vi "Init Drone.vi"() -> (1 "Video Interface":refnum<k16>, 2 "NavData Port":refnum<k16>, 3 "AT Command Port":refnum<k16>)   [LabVIEW 2011]
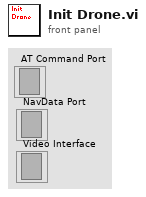
[diagram p1: front panel]
types:
  T1 = cluster{"Drone Status Bits":cluster{"Flying?":bool, "Video Enabled?":bool, "Vision Enabled?":bool, "Angular Speed Control?":bool, "Altitude Control?":bool, "Start button?":bool, "Control Command Recieved?":bool, "Trim Command Recieved?":bool, "Trim Running?":bool, "Trim Succeeded?":bool, "Navdata Demo Mode?":bool, "Navdata Bootstrap Mode?":bool, "Motors Com Down?":bool, "Unknown":bool, "Gyrometer Problem?":bool, "Battery Voltage Too Low?":bool, "Battery Voltage Too High?":bool, "Timer Elapsed?":bool, "Power Too Low?":bool, "Angles Out Of Range?":bool, "Too Much Wind?":bool, "Ultrasound Deaf?":bool, "Cutout Detected?":bool, "PIC Version Number OK?":bool, "ATCodec Thread On?":bool, "Navdata Thread On?":bool, "Video Thread On?":bool, "Acquisition Thread On?":bool, "Control Watchdog Delay?":bool, "ADC Watchdog Delay?":bool, "Communications Problem?":bool, "Emergency?":bool}, "Header":u32, "Sequence Number":u32, "Vision Defined?":bool, "Blocks":cluster{"Size":u16, "Data":u8[], "ID":enum16{"NAVDATA_DEMO", "NAVDATA_TIME", "NAVDATA_RAW_MEASURES", "NAVDATA_PHYS_MEASURES", "NAVDATA_GYROS_OFFSETS", "NAVDATA_EULER_ANGLES", "NAVDATA_REFERENCES", "NAVDATA_TRIMS", "NAVDATA_RC_REFERENCES", "NAVDATA_PWM", "NAVDATA_ALTITUDE", "NAVDATA_VISION_RAW", "NAVDATA_VISION_OF", "NAVDATA_VISION", "NAVDATA_VISION_PERF", "NAVDATA_TRACKERS_SEND", "NAVDATA_VISION_DETECT", "NAVDATA_WATCHDOG", "NAVDATA_ADC_DATA_FRAME", "NAVDATA_VIDEO_STREAM", "NAVDATA_GAMES"}}[]}
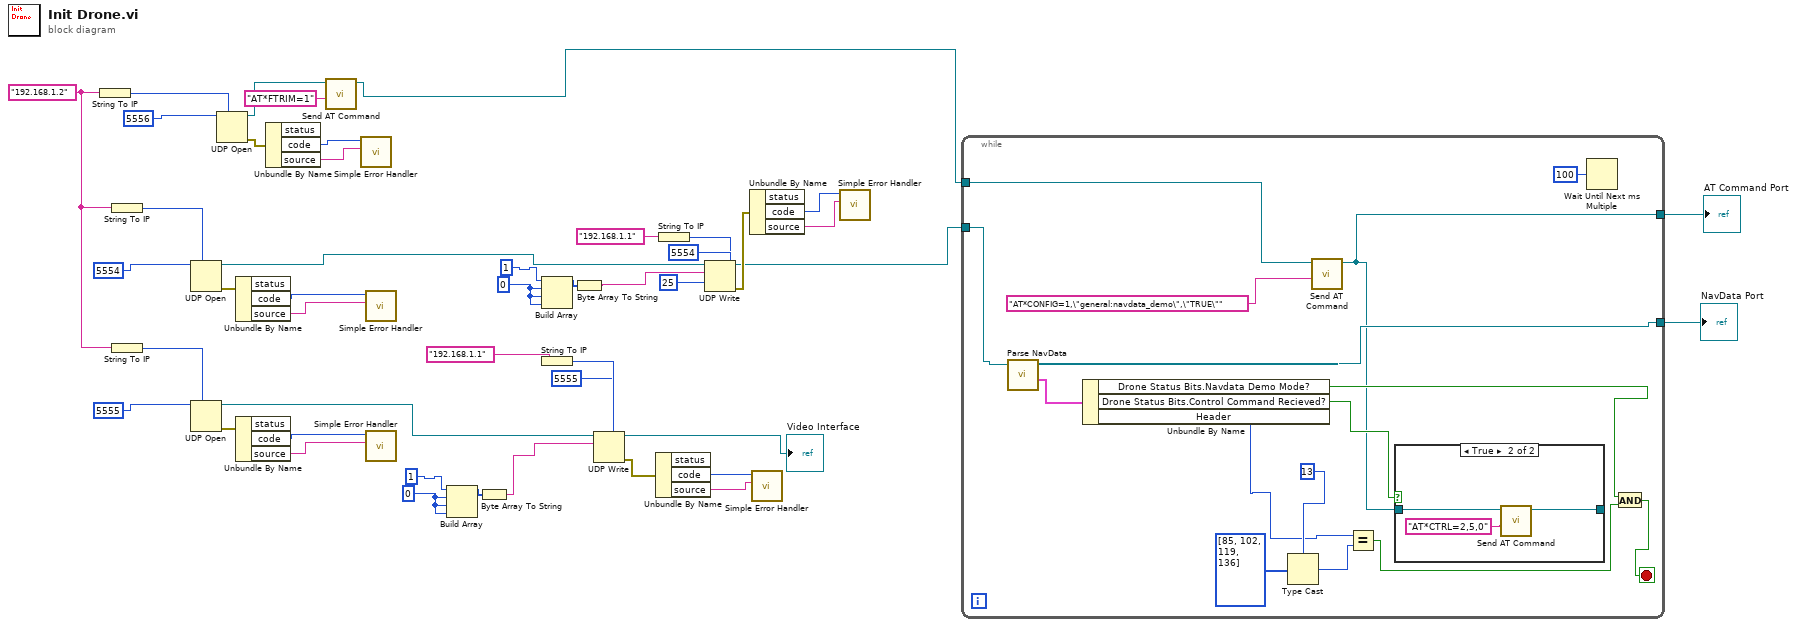
[diagram p0: block diagram]
diagram:
  w2 = u8 0
  w5 = u8 0
  w22 = "192.168.1.2"
  n1 = String To IP(1:w22) -> (0:w45:u32)
  n2 = String To IP(1:w22) -> (0:w43:u32)
  n3 = String To IP(1:w22) -> (0:w35:u32)
  n4 = UDP Open(7:w43, 11:u16 5554) -> (port=w10:refnum<k16>, 0:w42:errorcluster)  [unwired: 3 in, 1 out]
  n5 = UDP Open(7:w35, 11:u16 5555) -> (port=w26:refnum<k16>, 0:w34:errorcluster)  [unwired: 3 in, 1 out]
  n6 = UDP Open(7:w45, 11:u16 5556) -> (port=w21:refnum<k16>, 0:w39:errorcluster)  [unwired: 3 in, 1 out]
  n7 = Unbundle By Name(w42) -> ("code"=w41:i32, "source"=w40:string)  [unwired: 1 out]
  n8 = Unbundle By Name(w34) -> ("code"=w33:i32, "source"=w32:string)  [unwired: 1 out]
  n9 = Unbundle By Name(w39) -> ("code"=w38:i32, "source"=w37:string)  [unwired: 1 out]
  n10 = call "Send AT Command.vi"("AT Command"="AT*FTRIM=1", "AT Command Port"=w21) -> ("AT Command Port"=w19:refnum<k16>)  [unwired: 9 in]
  n11 = call <vilib>:"Simple Error Handler.vi"("error code (no error:0)"=w38, "error source (\" \")"=w37) -> ()  [unwired: 3 in, 5 out]
  n12 = call <vilib>:"Simple Error Handler.vi"("error code (no error:0)"=w41, "error source (\" \")"=w40) -> ()  [unwired: 3 in, 5 out]
  n13 = call <vilib>:"Simple Error Handler.vi"("error code (no error:0)"=w33, "error source (\" \")"=w32) -> ()  [unwired: 3 in, 5 out]
  n14 = Build Array(u8 1, w2, w2, w2) -> (w4:u8[])
  n15 = Byte Array To String(unsigned byte array=w4) -> (string=w1:string)
  n16 = Build Array(u8 1, w5, w5, w5) -> (w14:u8[])
  n17 = String To IP(1:"192.168.1.1") -> (0:w30:u32)
  n18 = Byte Array To String(unsigned byte array=w14) -> (string=w15:string)
  n19 = UDP Write(address=w30, port or service name=u16 5555, connection ID=w26, data in=w1) -> (error out=w28:errorcluster, 3:→"Video Interface":refnum<k16>)  [unwired: 2 in]
  n20 = Unbundle By Name(w28) -> ("code"=w24:i32, "source"=w25:string)  [unwired: 1 out]
  n21 = String To IP(1:"192.168.1.1") -> (0:w12:u32)
  n22 = UDP Write(address=w12, port or service name=u16 5554, connection ID=w10, data in=w15, 9:25) -> (error out=w16:errorcluster, 3:w7:refnum<k16>)  [unwired: 1 in]
  n23 = Unbundle By Name(w16) -> ("code"=w8:i32, "source"=w9:string)  [unwired: 1 out]
  n24 = call <vilib>:"Simple Error Handler.vi"("error code (no error:0)"=w24, "error source (\" \")"=w25) -> ()  [unwired: 3 in, 5 out]
  n25 = call <vilib>:"Simple Error Handler.vi"("error code (no error:0)"=w8, "error source (\" \")"=w9) -> ()  [unwired: 3 in, 5 out]
  n26 = while {
    tunnel: w19 -> [w52]
    tunnel: [w50] -> w23
    tunnel: w7 -> [w51]
    tunnel: [w49] -> w6
    stop <- w58 stop-if-true
    n27 = call "Parse NavData.vi"("NavData Port"=w51) -> ("NavData"=w48:T1, "NavData Port"=w50:refnum<k16>)  [unwired: 9 in]
    n28 = Unbundle By Name(w48) -> ("Drone Status Bits.Navdata Demo Mode?"=w59:bool, "Drone Status Bits.Control Command Recieved?"=w61:bool, "Header"=w47:u32)
    n29 = Type Cast(type=u32 13, x=u8[] [85, 102, 119, 136]) -> (*(type *) &x=w55:u32)
    n30 = call "Send AT Command.vi"("AT Command"="AT*CONFIG=1,\"general:navdata_demo\",\"TRUE\"", "AT Command Port"=w52) -> ("AT Command Port"=w49:refnum<k16>)  [unwired: 9 in]
    n31 = Equal?(x=w47, y=w55) -> (x = y?=w54:bool)
    n32 = case shown="True" w61 {
      tunnel: [w62 w64] -> _
      tunnel: w49 -> [w62 w63]
      frame False {
      }
      frame True {
        n33 = call "Send AT Command.vi"("AT Command"="AT*CTRL=2,5,0", "AT Command Port"=w63) -> ("AT Command Port"=w64:refnum<k16>)  [unwired: 9 in]
      }
    }
    n34 = Wait Until Next ms Multiple(millisecond multiple=u32 100) -> ()  [unwired: 1 out]
    n35 = And(x=w59, y=w54) -> (x .and. y?=w58:bool)
  }
  "AT Command Port" <- w6
  "NavData Port" <- w23
